vi "外观 1.vi"(0 "Data In":T4 caption="数据输入", 2 "Display State In":T2 caption="显示状态输入", 3 "Container State":T3 caption="容器状态") -> (6 "Data Out":T4 caption="数据输出", 7 "Display State Out":T2 caption="显示状态输出", 8 "Action":T1 caption="动作")   [LabVIEW 2019, in "运动轨迹控件.xctl"]
uses:
  <vilib>/_xctls/Container State.ctl
  <vilib>/_xctls/Action.ctl
  <vilib>/_xctls/XControlSupport.lvlib
panel:
  out "三维图片":refnum<vi>(3d-picture)
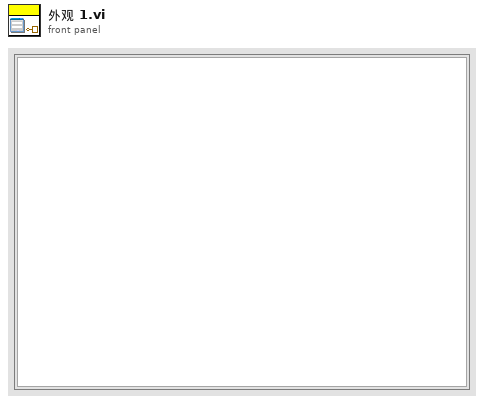
[diagram p1: front panel]
types:
  T1 = typedef "XControlSupport.lvlib/Action.ctl" = cluster{"Data Changed?":bool, "State Changed?":bool, "Action Name":string}
  T2 = typedef "运动轨迹控件.xctl/状态 1.ctl" = cluster{"刀具":cluster{"X":dbl, "Y":dbl, "Z":dbl}, "线段":cluster{"X":dbl, "Y":dbl, "Z":dbl}}
  T3 = typedef "XControlSupport.lvlib/Container State.ctl" = cluster{"Indicator?":bool, "Run Mode?":bool, " Refnum":refnum<vi>}
  T4 = typedef "运动轨迹控件.xctl/数据 1.ctl" = cluster{"X":dbl, "Y":dbl, "Z":dbl}[]
  T5 = enum16{"None", "Spherical", "Flying", "Oriented"}
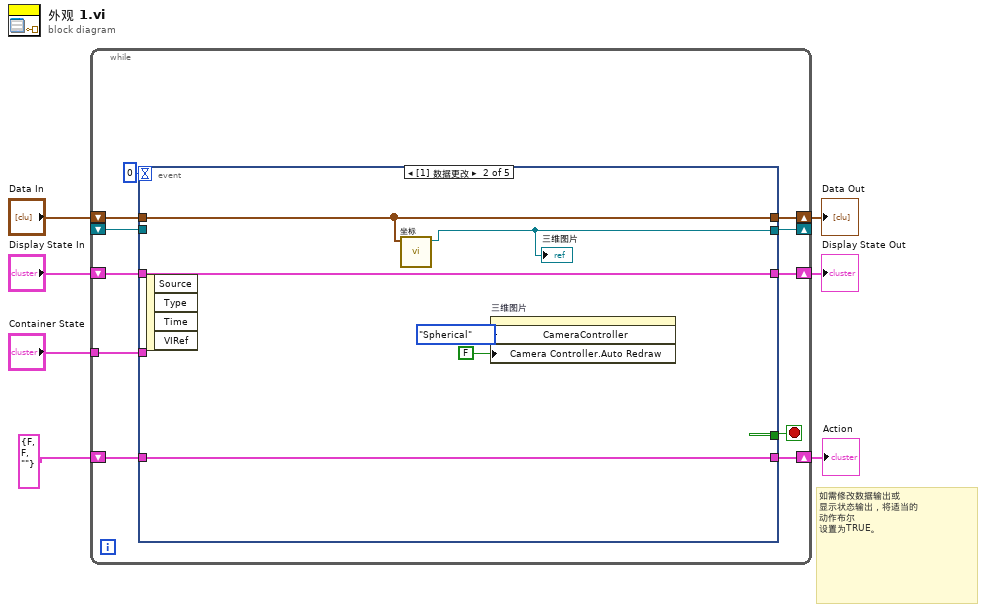
[diagram p0: block diagram]
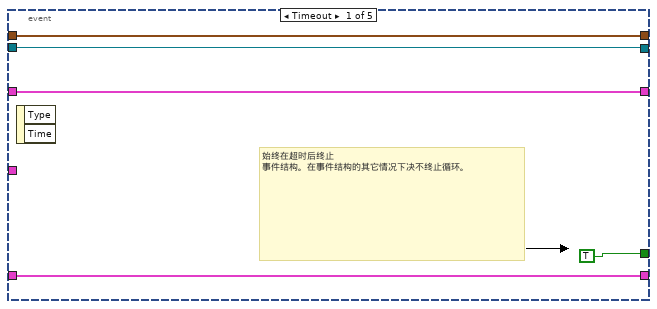
[diagram p2: hidden frame]
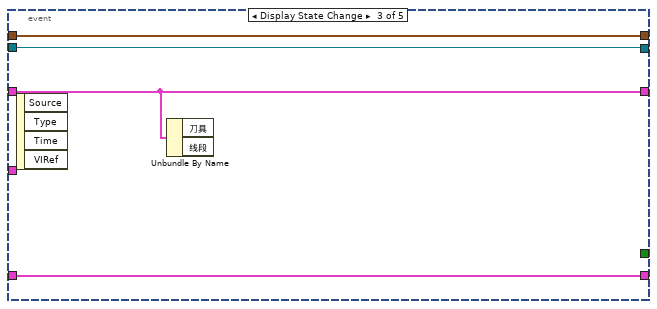
[diagram p3: hidden frame]
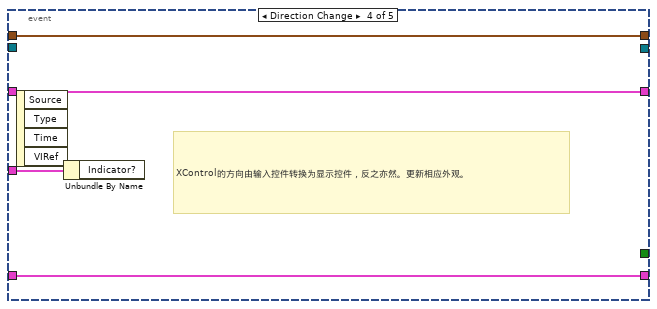
[diagram p4: hidden frame]
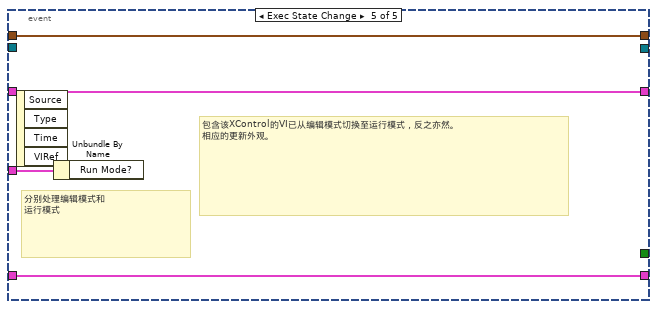
[diagram p5: hidden frame]
diagram:
  # "如需修改数据输出或\n显示状态输出，将适当的\n动作布尔\n设置为TRUE。"
  n1 = while {
    shift-right: [w17] -> w4
    shift-left: "Display State In" -> [w18]
    tunnel: "Container State" -> [w14]
    shift-right: [w12] -> w7
    shift-left: "Data In" -> [w13]
    shift-right: [w10] -> w2
    shift-left: T1 {"Data Changed?"=FALSE, "State Changed?"=FALSE, "Action Name"=""} ("Action") -> [w11]
    shift-right: [w8] -> _
    shift-left: _ -> [w9]
    stop <- w16 stop-if-true
    n2 = event shown="[1] 数据更改" {
      selector: _ -> [_ _ _ _ _]
      dyn-events: _ -> [_ _ _ _ _]
      timeout: 0 -> [_ _ _ _ _]
      tunnel: w18 -> [w21 w26 w31 w36 w40]
      tunnel: [w21 w26 w31 w36 w40] -> w17
      tunnel: [TRUE _ _ _ _] -> w16
      tunnel: w14 -> [_ _ _ w37 w41]
      tunnel: w13 -> [w20 w28 w33 w35 w39]
      tunnel: [w20 w28 w33 w35 w39] -> w12
      tunnel: [w22 w29 w32 w34 w38] -> w10
      tunnel: w11 -> [w22 w29 w32 w34 w38]
      tunnel: [w19 w27 w30 _ _] -> w8
      tunnel: w9 -> [w19 _ w30 _ _]
      event Timeout {
        # "始终在超时后终止\n事件结构。在事件结构的其它情况下决不终止循环。"
        n3 = event-data() -> ()  [unwired: 1 in, 2 out]
      }
      event Data Change {
        n4 = event-data() -> ()  [unwired: 1 in, 4 out]
        n5 = call "坐标.vi"("线段"=w28) -> ("Scene Object Out"=w27:refnum<vi>)  [unwired: 8 in, 1 out]
        "三维图片" <- w27
        n6 = property on="三维图片" class="SceneGraphDisp (严格)"("CameraController"=T5."Spherical" ("视角控制器:类型"), "Camera Controller.Auto Redraw"=FALSE ("视角控制器:自动重绘")) -> ()  [unwired: 2 in, 2 out]
      }
      event Display State Change {
        n7 = event-data() -> ()  [unwired: 1 in, 4 out]
        n8 = Unbundle By Name(w31) -> ()  [unwired: 2 out]
      }
      event Direction Change {
        # "XControl的方向由输入控件转换为显示控件，反之亦然。更新相应外观。"
        n9 = event-data() -> ()  [unwired: 1 in, 4 out]
        n10 = Unbundle By Name(w37) -> ()  [unwired: 1 out]
      }
      event Exec State Change {
        # "包含该XControl的VI已从编辑模式切换至运行模式，反之亦然。\n相应的更新外观。"
        # "分别处理编辑模式和\n运行模式"
        n11 = event-data() -> ()  [unwired: 1 in, 4 out]
        n12 = Unbundle By Name(w41) -> ()  [unwired: 1 out]
      }
    }
  }
  "Display State Out" <- w4
  "Data Out" <- w7
  "Action" <- w2
